vi "VI Get All Output.vi"(8 "error in (no error)":errorcluster, 11 "CallVIStep in":refnum<class "CallVIStep.lvclass">) -> (0 "error out":errorcluster, 2 "Output":T1[](array[typedef]), 3 "CallVIStep out":refnum<class "CallVIStep.lvclass">)   [LabVIEW 2015, in "CallVIStep.lvclass"]
uses:
  CallVIStep.lvclass
  Step/STEP_OUTPUT.ctl
  Step/OUTPUT_DATA_TYPE.ctl
  OutputUI/OUTPUT_CHECK_TYPE.ctl
  Step/OUTPUT_VALUE_TYPE.ctl
  Step.lvclass
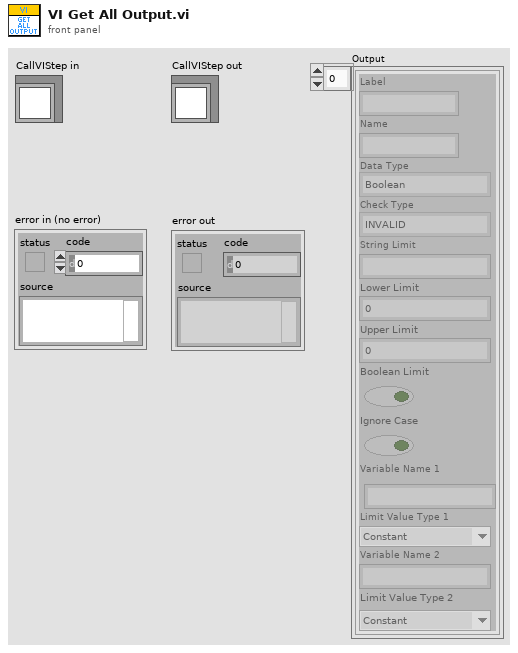
[diagram p1: front panel]
types:
  T1 = typedef "Step.lvclass/STEP_OUTPUT.ctl" = cluster{"Label":string, "Name":string, "Data Type":T2, "Check Type":T3, "String Limit":string, "Lower Limit":dbl, "Upper Limit":dbl, "Boolean Limit":bool, "Ignore Case":bool, "Variable Name 1":string, "Limit Value Type 1":T4, "Variable Name 2":string, "Limit Value Type 2":T4}
  T2 = typedef "Step.lvclass/OUTPUT_DATA_TYPE.ctl" = enum16{"Boolean", "String", "Numeric", "Other"}
  T3 = typedef "Step.lvclass/OUTPUT_CHECK_TYPE.ctl" = enum16{"INVALID", "DO_NOT_CHECK", "RECORD", "VARIABLE", "EQUAL", "NOT_EQUAL", "STR_CONTAINS", "STR_START_WITH", "STR_END_WITH", "STR_REGEX_MATCH", "NUM_GT", "NUM_LT", "NUM_GE", "NUM_LE", "NUM_RANGE", "NUM_RANGE_BDY"}
  T4 = typedef "Step.lvclass/OUTPUT_VALUE_TYPE.ctl" = enum16{"Constant", "Variable"}
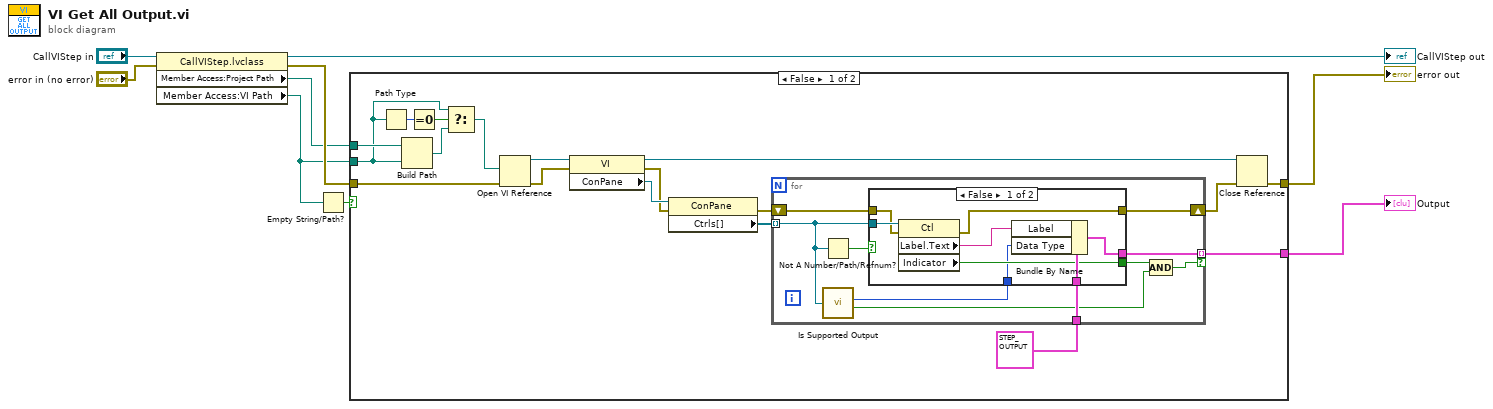
[diagram p0: block diagram]
diagram:
  n1 = property class="CallVIStep.lvclass"(reference="CallVIStep in", error in="error in (no error)") -> (reference out=→"CallVIStep out":refnum<class "CallVIStep.lvclass">, error out=w9:errorcluster, "Member Access:Project Path"=w2:path, "Member Access:VI Path"=w1:path)
  n2 = Empty String/Path?(string/path=w1) -> (empty?=w8:bool)
  n3 = case shown="False" w8 {
    tunnel: w9 -> [w27 w47]
    tunnel: [w19 _] -> w3
    tunnel: w1 -> [w12 _]
    tunnel: [w17 w47] -> w4
    tunnel: w2 -> [w15 _]
    frame False {
      n4 = Path Type(1:w12) -> (0:w14:i16)
      n5 = Build Path(base path=w15, name or relative path=w12) -> (appended path=w11:path)
      n6 = Equal To 0?(x=w14) -> (x = 0?=w13:bool)
      n7 = Select(t=w12, s=w13, f=w11) -> (s? t:f=w10:path)
      n8 = Open VI Reference(vi path=w10, error in (no error)=w27) -> (vi reference=w23:refnum<vi>, error out=w22:errorcluster)  [unwired: 4 in]
      n9 = property class="VI"(reference=w23, error in=w22) -> (reference out=w26:refnum<vi>, error out=w21:errorcluster, "ConPane"=w25:refnum<vi>)
      n10 = property class="ConPane"(reference=w25, error in=w21) -> (error out=w20:errorcluster, "Ctrls[]"=w24:refnum<vi>[])  [unwired: 1 out]
      n11 = for {
        tunnel: w24 -> [w30] mode=indexing
        tunnel: [w35] -> w19 mode=indexing if=w34
        shift-right: [w31] -> w18
        shift-left: w20 -> [w33]
        tunnel: T1 {"Label"="", "Name"="", "Data Type"=enum."Boolean", "Check Type"=enum."DO_NOT_CHECK", "String Limit"="", "Lower Limit"=0.0, "Upper Limit"=0.0, "Boolean Limit"=FALSE, "Ignore Case"=FALSE, "Variable Name 1"="", "Limit Value Type 1"=enum."Constant", "Variable Name 2"="", "Limit Value Type 2"=enum."Constant"} -> [w32]
        n12 = Not A Number/Path/Refnum?(number/path/refnum=w30) -> (NaN/Path/Refnum?=w36:bool)
        n13 = call "Is Supported Output.vi"("Ctl Refnum"=w30) -> ("Type"=w28:T2, "Supported"=w29:bool)  [unwired: 8 in]
        n14 = case shown="False" w36 {
          tunnel: w30 -> [w45 _]
          tunnel: [w44 _] -> w35
          tunnel: [w40 _] -> w37
          tunnel: w33 -> [w43 w46]
          tunnel: w32 -> [w42 _]
          tunnel: [w41 w46] -> w31
          tunnel: w28 -> [w38 _]
          frame False {
            n15 = property class="Ctl"(reference=w45, error in=w43) -> (error out=w41:errorcluster, "Label.Text"=w39:string, "Indicator"=w40:bool)  [unwired: 1 out]
            n16 = Bundle By Name(cluster=w42, "Label"=w39, "Data Type"=w38) -> (w44:T1)
          }
          frame True {
          }
        }
        n17 = Compound Arithmetic op=AND(w37, w29) -> (w34:bool)
      }
      n18 = Close Reference(reference=w26, error in (no error)=w18) -> (error out=w17:errorcluster)
    }
    frame True {
    }
  }
  "error out" <- w4
  "Output" <- w3
